vi "GetAccelerometerDataField.vi"(10 "Telemetry Data":string, 11 "Cluster in":refnum<vi>) -> (3 "Array":string[](array[string]))   [LabVIEW 2016]
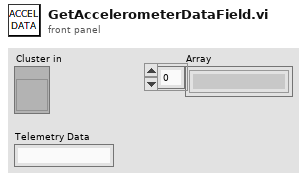
[diagram p1: front panel]
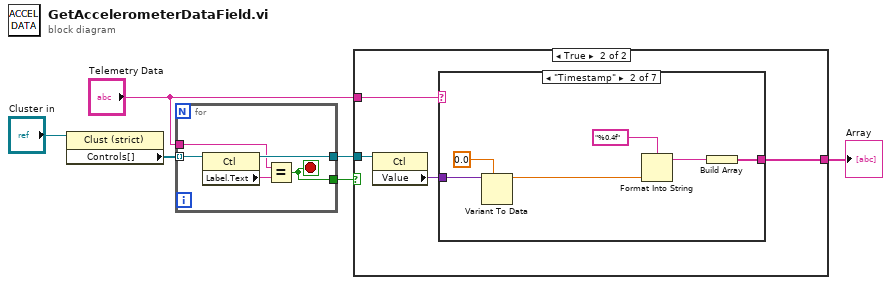
[diagram p0: block diagram]
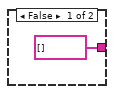
[diagram p2: hidden frame]
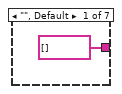
[diagram p3: hidden frame]
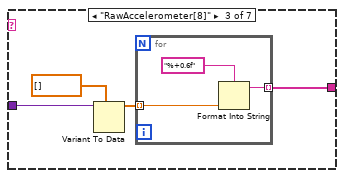
[diagram p4: hidden frame]
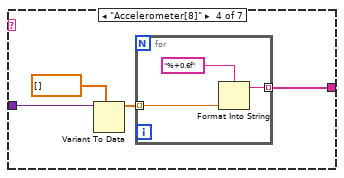
[diagram p5: hidden frame]
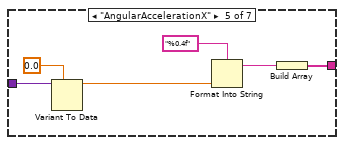
[diagram p6: hidden frame]
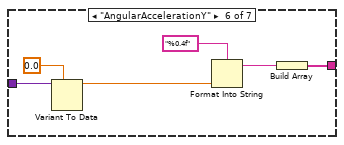
[diagram p7: hidden frame]
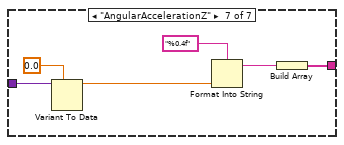
[diagram p8: hidden frame]
diagram:
  n1 = property on="Property Node" class="Clust (strict)"(reference="Cluster in") -> ("Controls[]"=w6:refnum<vi>[])  [unwired: 1 in, 2 out]
  n2 = for {
    tunnel: w6 -> [w11] mode=indexing
    tunnel: [w10] -> w1
    tunnel: "Telemetry Data" -> [w8]
    tunnel: [w7] -> w2
    stop <- w7 stop-if-true
    n3 = property on="Property Node" class="Ctl"(reference=w11) -> (reference out=w10:refnum<vi>, "Label.Text"=w9:string)  [unwired: 1 in, 1 out]
    n4 = Equal?(x=w8, y=w9) -> (x = y?=w7:bool)
  }
  n5 = case shown="True" w2 {
    tunnel: "Telemetry Data" -> [_ w16]
    tunnel: w1 -> [_ w15]
    tunnel: [string[] [] w13] -> w4
    frame False {
    }
    frame True {
      n6 = property on="Property Node" class="Ctl"(reference=w15) -> ("Value"=w14:variant)  [unwired: 1 in, 2 out]
      n7 = case shown="\"Timestamp\"" w16 {
        tunnel: [string[] [] w21 w24 w31 w41 w47 w53] -> w13
        tunnel: w14 -> [_ w19 w27 w34 w39 w45 w51]
        frame "", Default {
        }
        frame "Timestamp" {
          n8 = Variant To Data(type=0.0, Variant=w19) -> (data=w20:dbl)  [unwired: 1 in, 1 out]
          n9 = Format Into String(format string="%0.4f", w20) -> (resulting string=w22:string)  [unwired: 2 in, 1 out]
          n10 = Build Array(w22) -> (w21:string[])
        }
        frame "RawAccelerometer[8]" {
          n11 = Variant To Data(type=sgl[] [], Variant=w27) -> (data=w25:sgl[])  [unwired: 1 in, 1 out]
          n12 = for {
            tunnel: w25 -> [w29] mode=indexing
            tunnel: [w28] -> w24 mode=indexing
            n13 = Format Into String(format string="%+0.6f", w29) -> (resulting string=w28:string)  [unwired: 2 in, 1 out]
          }
        }
        frame "Accelerometer[8]" {
          n14 = Variant To Data(type=sgl[] [], Variant=w34) -> (data=w32:sgl[])  [unwired: 1 in, 1 out]
          n15 = for {
            tunnel: w32 -> [w36] mode=indexing
            tunnel: [w35] -> w31 mode=indexing
            n16 = Format Into String(format string="%+0.6f", w36) -> (resulting string=w35:string)  [unwired: 2 in, 1 out]
          }
        }
        frame "AngularAccelerationX" {
          n17 = Variant To Data(type=0.0, Variant=w39) -> (data=w40:dbl)  [unwired: 1 in, 1 out]
          n18 = Format Into String(format string="%0.4f", w40) -> (resulting string=w42:string)  [unwired: 2 in, 1 out]
          n19 = Build Array(w42) -> (w41:string[])
        }
        frame "AngularAccelerationY" {
          n20 = Variant To Data(type=0.0, Variant=w45) -> (data=w46:dbl)  [unwired: 1 in, 1 out]
          n21 = Format Into String(format string="%0.4f", w46) -> (resulting string=w48:string)  [unwired: 2 in, 1 out]
          n22 = Build Array(w48) -> (w47:string[])
        }
        frame "AngularAccelerationZ" {
          n23 = Variant To Data(type=0.0, Variant=w51) -> (data=w52:dbl)  [unwired: 1 in, 1 out]
          n24 = Format Into String(format string="%0.4f", w52) -> (resulting string=w54:string)  [unwired: 2 in, 1 out]
          n25 = Build Array(w54) -> (w53:string[])
        }
      }
    }
  }
  "Array" <- w4
